vi "Check-Uncheck.vi"(8 "Enabled out":bool[](array[boolean]), 9 "Coords":T1, 11 "Listbox Ref":refnum<vi>) -> (0 "Enabled in":bool[](array[boolean]))   [LabVIEW 2017]
uses:
  <vilib>/Utility/miscctls.llb/LVPoint32TypeDef.ctl
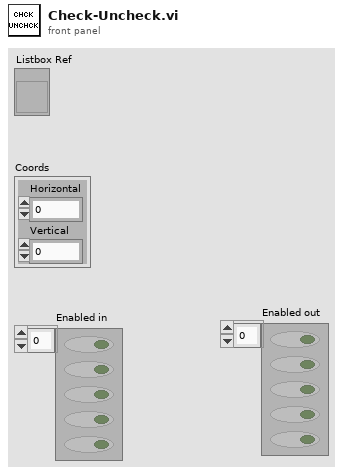
[diagram p1: front panel]
types:
  T1 = typedef "LVPoint32TypeDef.ctl" = cluster{"Horizontal":i32, "Vertical":i32}
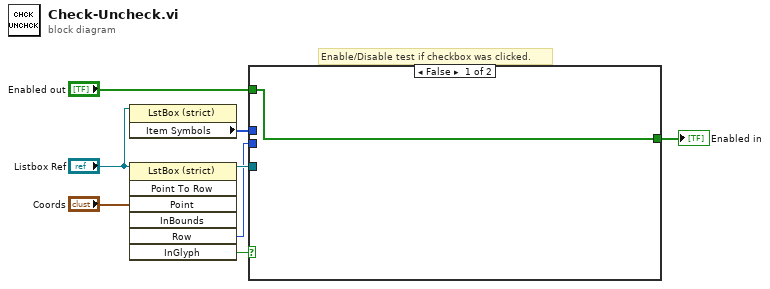
[diagram p0: block diagram]
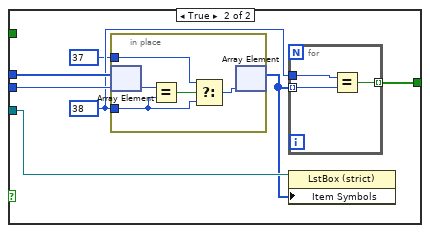
[diagram p2: hidden frame]
diagram:
  # "Enable/Disable test if checkbox was clicked."
  n1 = property on="Property Node" class="LstBox (strict)"(reference="Listbox Ref") -> ("Item Symbols"=w7:i32[])  [unwired: 1 in, 2 out]
  n2 = invoke on="Invoke Node" class="LstBox (strict)" method="Point To Row"(reference="Listbox Ref", "Point"="Coords") -> (reference out=w8:refnum<vi>, "Row"=w3:i32, "InGlyph"=w6:bool)  [unwired: 5 in, 4 out]
  n3 = case shown="False" w6 {
    tunnel: w3 -> [_ w15]
    tunnel: w7 -> [_ w16]
    tunnel: "Enabled out" -> [w9 _]
    tunnel: [w9 w10] -> w1
    tunnel: w8 -> [_ w14]
    frame False {
    }
    frame True {
      w12 = 38
      n4 = in-place "In Place Element Structure" {
        in-place-border: 37 -> [w23]
        in-place-border: w12 -> [w22]
        n5 = in-place-array #1 ("Array Index / Replace Elements")(w16, w15) -> (w21:i32)
        n6 = Equal?(x=w21, y=w22) -> (x = y?=w24:bool)
        n7 = Select(t=w23, s=w24, f=w22) -> (s? t:f=w20:i32)
        n8 = in-place-array #1 ("Array Index / Replace Elements")(w20) -> (w13:i32[])  [unwired: 1 out]
      }
      n9 = for {
        tunnel: w13 -> [w18] mode=indexing
        tunnel: [w19] -> w10 mode=indexing
        tunnel: w12 -> [w17]
        n10 = Equal?(x=w17, y=w18) -> (x = y?=w19:bool)
      }
      n11 = property on="Property Node" class="LstBox (strict)"(reference=w14, "Item Symbols"=w13) -> ()  [unwired: 1 in, 2 out]
    }
  }
  "Enabled in" <- w1
